vi "Config Type Def to Generic Type Defs.vi"(11 "measurement configuration":T15={"digital serial cfg file"="", "digital channel list"="7821\\PCMo 8", "master clock channel list"="7821\\PCMo 0", "output level"=-1.0, "output level units"=enum."dBFS", "output range (pk-pk)"=15.0, "load impedance"=4.0, "signal phase"=0.0, "acq sampling rate"=51200.0, "min measurement cycles"=20, "min measurement time (s)"=0.1, "min settling cycles"=0, "min settling time (s)"=0.0, "acq channel"="", "band start"=20.0, "band stop"=20000.0, "weighting filter"=enum."A-weighting", "highpass filter"=enum."DC", "lowpass filter"=enum."No filter", "sweep start frequency (Hz)"=20.0, "sweep stop frequency (Hz)"=20000.0, "number of steps"=10, "sweep profile"=enum."Logarithmic", "SNR units"=enum."dB", "THD+N units"=enum."dB", "THD units"=enum."dB", "gain units"=enum."dB", "enable regulation"=FALSE, "regulation target"=enum."THD+N Ratio", "regulation target value"=0.05, "regulation target value units"=enum."%", "regulation start level"=10.0, "regulation stop level"=70.0, "regulation number of steps"=2} {"min settling cycles" format="%#_6pHz"; "sweep start frequency (Hz)" format="%0.2f"; "acq sampling rate" format="%0.2f"}) -> (2 "regulation settings":T12={"enable regulation"=FALSE, "regulation target"=enum."THD+N Ratio", "regulation target value"=0.05, "regulation target value units"=enum."%", "regulation start level"=10.0, "regulation stop level"=70.0, "regulation number of steps"=2}, 3 "single tone settings":T1={"digital channel list"="7821\\PCMo 8", "frame clock rate"=48000.0, "number of channels"=2, "channel length"=32, "bit depth"=24, "data justification"=enum."Left Justified", "endianness"=enum."MSB First", "bit clock edge sync"=enum."Falling", "frame sync edge for channel 0"=enum."Falling", "channel 0 offset"=1, "master clock channel list"="7821\\PCMo 0", "master clock rate"=12288000.0, "enable dither"=TRUE, "logic level"=enum."3.3 V", "signal frequency"=1000.0, "output level"=-1.0, "output level units"=enum."dBFS", "output range (pk-pk)"=15.0, "load impedance"=4.0, "signal phase"=0.0, "acq sampling rate"=51200.0, "min measurement cycles"=20, "min measurement time (s)"=0.1, "min settling cycles"=0, "min settling time (s)"=0.0, "acq channel"="", "band start"=20.0, "band stop"=20000.0, "weighting filter"=enum."A-weighting", "highpass filter"=enum."DC", "lowpass filter"=enum."No filter", "SNR units"=enum."dB", "THD+N units"=enum."dB", "THD units"=enum."dB", "gain units"=enum."dB"} {"signal phase" format="%0.2f"; "master clock rate" format="%#_6pHz"; "frame clock rate" format="%#_6pHz"})   [LabVIEW 2021, in "Stepped Frequency Sweep_Class D Amplifier.lvlib"]
uses:
  Stepped Frequency Sweep_Class D Amplifier.lvlib
  Measurement Configuration.ctl
  shared/controls/digital output level units.ctl
  shared/controls/weighting filter.ctl
  shared/controls/highpass filter.ctl
  shared/controls/lowpass filter.ctl
  shared/controls/sweep profile.ctl
  shared/controls/units - snr.ctl
  shared/controls/units - ratio.ctl
  shared/controls/regulation target.ctl
  shared/controls/regulation target value units.ctl
  shared/controls/regulation settings.ctl
  shared/controls/single tone measurement settings (HW).ctl
  shared/controls/digital audio protocol/data justification.ctl
  shared/controls/digital audio protocol/endianness.ctl
  shared/controls/digital audio protocol/digital edge.ctl
  shared/controls/digital audio protocol/logic level.ctl
  shared/controls/audio controls.lvlib
  shared/digital serial gen settings/digital audio protocol controls.lvlib
panel:
  out "error out":errorcluster
  in  "error in (no error)":errorcluster
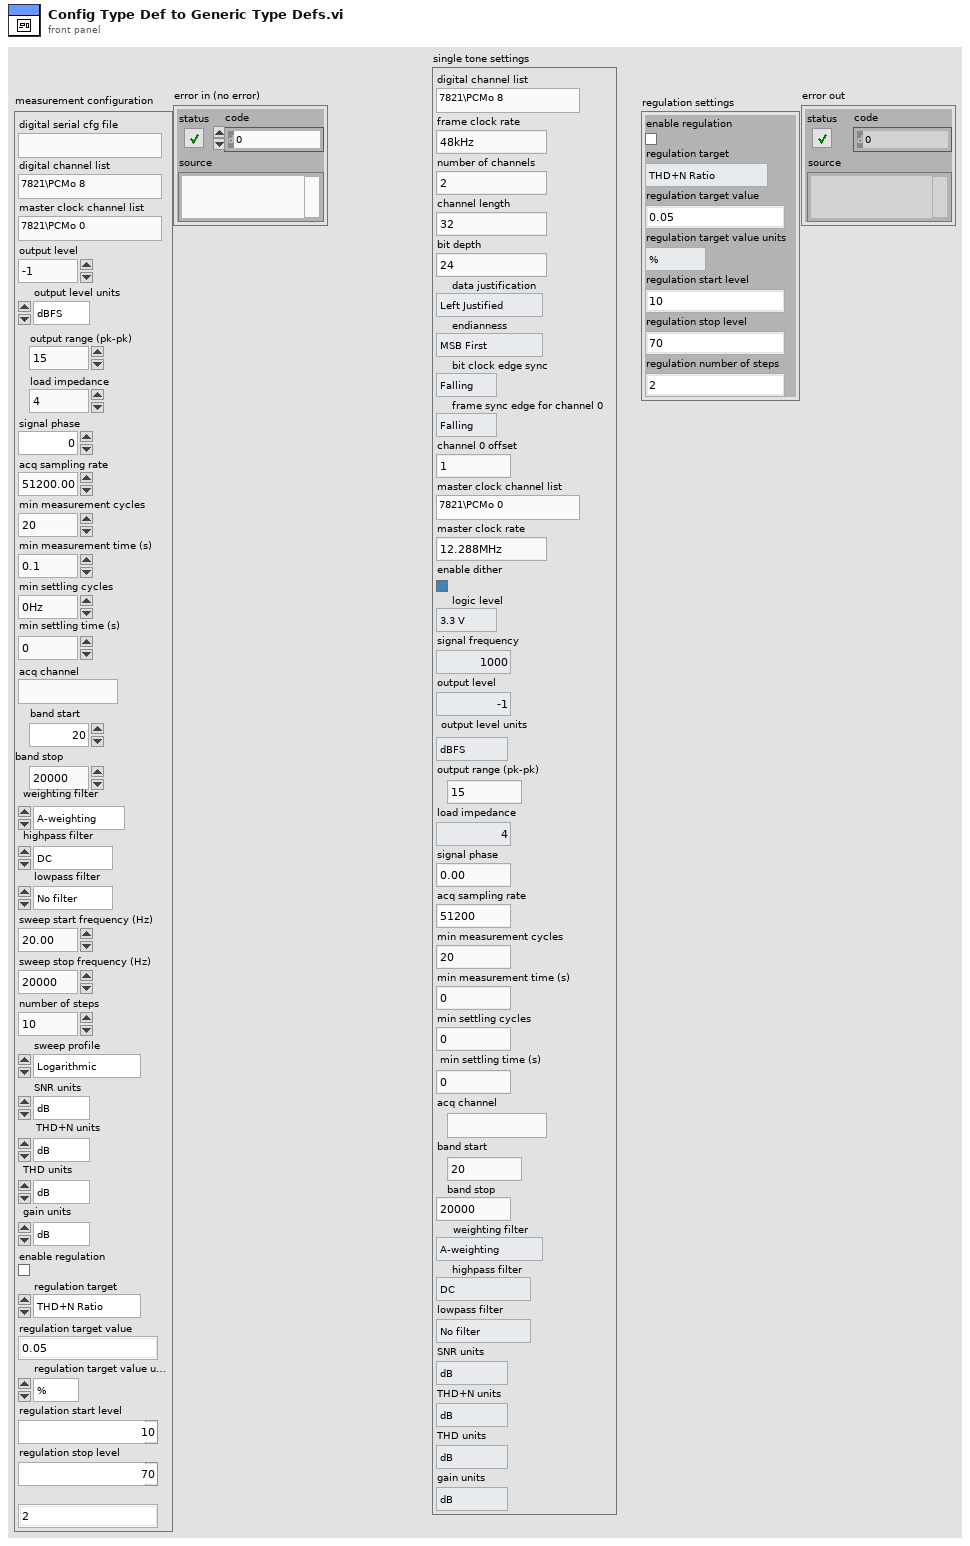
[diagram p1: front panel]
types:
  T1 = typedef "single tone measurement settings (HW).ctl" = cluster{"digital channel list":string, "frame clock rate":dbl, "number of channels":u32, "channel length":u32, "bit depth":u32, "data justification":T2, "endianness":T3, "bit clock edge sync":T4, "frame sync edge for channel 0":T4, "channel 0 offset":u32, "master clock channel list":string, "master clock rate":dbl, "enable dither":bool, "logic level":T5, "signal frequency":dbl, "output level":dbl, "output level units":T6, "output range (pk-pk)":dbl, "load impedance":dbl, "signal phase":dbl, "acq sampling rate":dbl, "min measurement cycles":u32, "min measurement time (s)":dbl, "min settling cycles":u32, "min settling time (s)":dbl, "acq channel":string, "band start":dbl, "band stop":dbl, "weighting filter":T7, "highpass filter":T8, "lowpass filter":T9, "SNR units":T10, "THD+N units":T11, "THD units":T11, "gain units":T11}
  T2 = typedef "data justification.ctl" = enum32{"Left Justified", "Right Justified"}
  T3 = typedef "endianness.ctl" = enum32{"MSB First", "LSB First"}
  T4 = typedef "digital edge.ctl" = enum32{"Rising", "Falling"}
  T5 = typedef "logic level.ctl" = enum32{"3.3 V", "1.8 V", "1.2 V"}
  T6 = typedef "audio controls.lvlib/digital output level units.ctl" = enum32{"% FS", "dBFS", "V"}
  T7 = typedef "weighting filter.ctl" = enum32{"Linear", "A-weighting", "B-weighting", "C-weighting"}
  T8 = typedef "highpass filter.ctl" = enum32{"DC", "AC"}
  T9 = typedef "lowpass filter.ctl" = enum32{"No filter", "AES17 20kHz", "AES17 40kHz"}
  T10 = typedef "audio controls.lvlib/units - snr.ctl" = enum32{"dB", "x/y"}
  T11 = typedef "audio controls.lvlib/units - ratio.ctl" = enum32{"dB", "%", "x/y"}
  T12 = typedef "regulation settings.ctl" = cluster{"enable regulation":bool, "regulation target":T13, "regulation target value":dbl, "regulation target value units":T14, "regulation start level":dbl, "regulation stop level":dbl, "regulation number of steps":u32}
  T13 = typedef "regulation target.ctl" = enum32{"THD+N Ratio", "Output Power"}
  T14 = typedef "regulation target value units.ctl" = enum32{"%", "W"}
  T15 = typedef "Stepped Frequency Sweep_Class D Amplifier.lvlib/Measurement Configuration.ctl" = cluster{"digital serial cfg file":string, "digital channel list":string, "master clock channel list":string, "output level":dbl, "output level units":T6, "output range (pk-pk)":dbl, "load impedance":dbl, "signal phase":dbl, "acq sampling rate":dbl, "min measurement cycles":u32, "min measurement time (s)":dbl, "min settling cycles":u32, "min settling time (s)":dbl, "acq channel":string, "band start":dbl, "band stop":dbl, "weighting filter":T7, "highpass filter":T8, "lowpass filter":T9, "sweep start frequency (Hz)":dbl, "sweep stop frequency (Hz)":dbl, "number of steps":u32, "sweep profile":T16, "SNR units":T10, "THD+N units":T11, "THD units":T11, "gain units":T11, "enable regulation":bool, "regulation target":T13, "regulation target value":dbl, "regulation target value units":T14, "regulation start level":dbl, "regulation stop level":dbl, "regulation number of steps":u32}
  T16 = typedef "audio controls.lvlib/sweep profile.ctl" = enum32{"Linear", "Logarithmic"}
  T17 = typedef "digital serial gen settings.ctl" = cluster{"number of channels":u32, "data justification":T18, "endianness":T19, "channel length":u32, "bit depth":u32, "frame clock rate":dbl, "bit clock edge sync":T20, "master clock rate":dbl, "Logic Level":T21, "frame sync edge for channel 0":T20, "Channel 0 Offset":u32}
  T18 = typedef "PDM Shared.lvlib/PCM Data Justification.ctl" = enum16{"Left Justified", "Right Justified"}
  T19 = typedef "PDM Shared.lvlib/PCM Bit Endianness.ctl" = enum16{"MSB First", "LSB First"}
  T20 = typedef "PDM Shared.lvlib/Digital Edge.ctl" = enum8{"Rising", "Falling"}
  T21 = typedef "PDM Acquisition Class Library.lvlib/DecoderSession.lvclass/Logic Levels.ctl" = enum16{"3.3 V", "1.8 V", "1.2 V"}
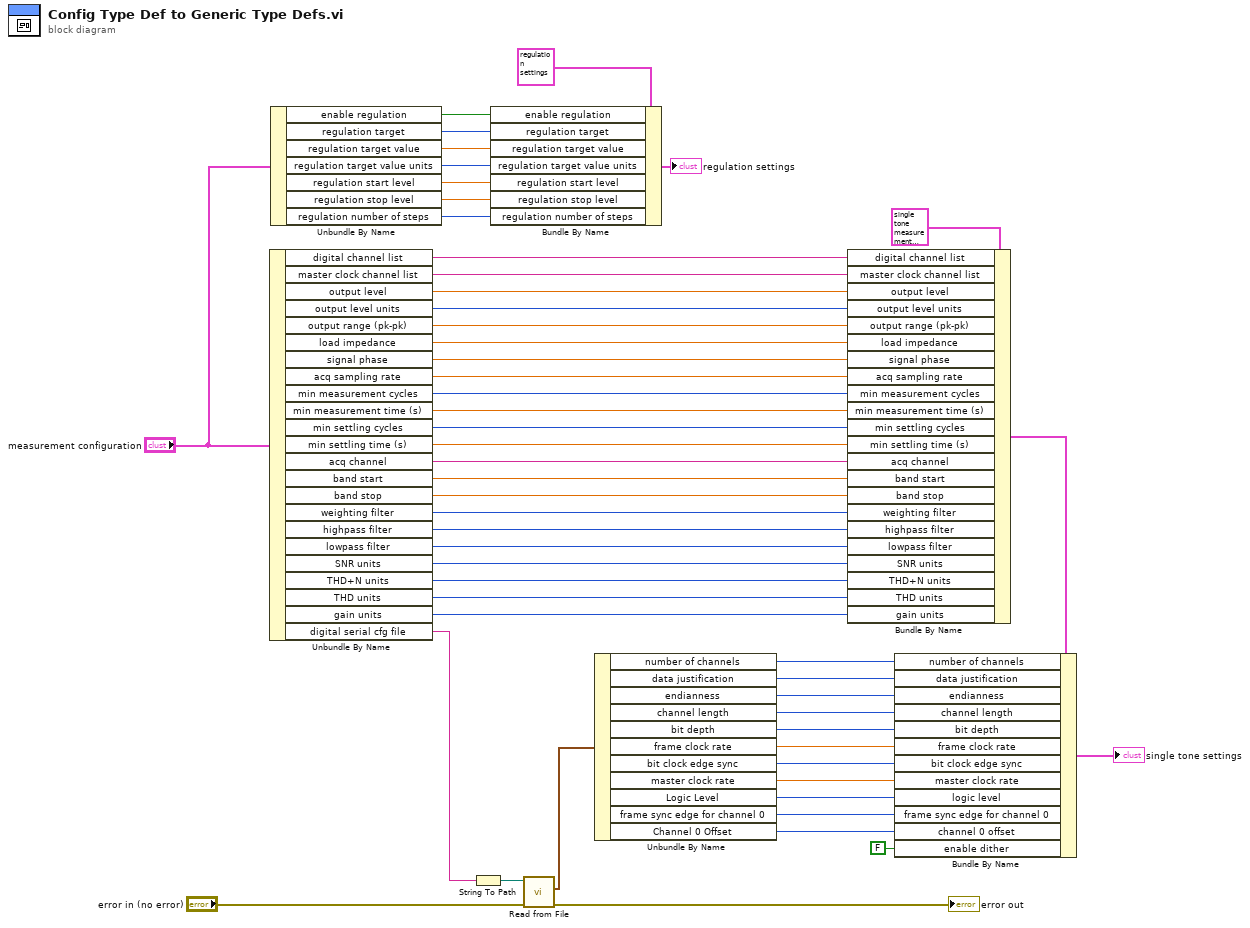
[diagram p0: block diagram]
diagram:
  n1 = Unbundle By Name("measurement configuration") -> ("digital channel list"=w42:string, "master clock channel list"=w41:string, "output level"=w21:dbl, "output level units"=w40:T6, "output range (pk-pk)"=w39:dbl, "load impedance"=w38:dbl, "signal phase"=w37:dbl, "acq sampling rate"=w36:dbl, "min measurement cycles"=w35:u32, "min measurement time (s)"=w34:dbl, "min settling cycles"=w33:u32, "min settling time (s)"=w32:dbl, "acq channel"=w31:string, "band start"=w30:dbl, "band stop"=w29:dbl, "weighting filter"=w28:T7, "highpass filter"=w27:T8, "lowpass filter"=w26:T9, "SNR units"=w25:T10, "THD+N units"=w24:T11, "THD units"=w23:T11, "gain units"=w22:T11, "digital serial cfg file"=w18:string)
  n2 = Unbundle By Name("measurement configuration") -> ("enable regulation"=w51:bool, "regulation target"=w50:T13, "regulation target value"=w49:dbl, "regulation target value units"=w48:T14, "regulation start level"=w47:dbl, "regulation stop level"=w46:dbl, "regulation number of steps"=w45:u32)
  n3 = String To Path(string=w18) -> (path=w20:path)
  n4 = Bundle By Name(cluster=T12 {"enable regulation"=FALSE, "regulation target"=enum."THD+N Ratio", "regulation target value"=0.05, "regulation target value units"=enum."%", "regulation start level"=10.0, "regulation stop level"=70.0, "regulation number of steps"=2} ("regaultion settings"), "enable regulation"=w51, "regulation target"=w50, "regulation target value"=w49, "regulation target value units"=w48, "regulation start level"=w47, "regulation stop level"=w46, "regulation number of steps"=w45) -> (→"regulation settings":T12)
  n5 = call "Read from File.vi"("error in (no error)"="error in (no error)", "file path"=w20) -> ("error out"=→"error out":errorcluster, "digital audio protocol settings"=w16:T17)  [unwired: 7 in, 1 out]
  n6 = Unbundle By Name(w16) -> ("number of channels"=w14:u32, "data justification"=w12:T18, "endianness"=w11:T19, "channel length"=w10:u32, "bit depth"=w9:u32, "frame clock rate"=w8:dbl, "bit clock edge sync"=w7:T20, "master clock rate"=w6:dbl, "Logic Level"=w5:T21, "frame sync edge for channel 0"=w4:T20, "Channel 0 Offset"=w3:u32)
  n7 = Bundle By Name(cluster=T1 {"digital channel list"="7821\\PCMo 8", "frame clock rate"=48000.0, "number of channels"=2, "channel length"=32, "bit depth"=24, "data justification"=enum."Left Justified", "endianness"=enum."MSB First", "bit clock edge sync"=enum."Falling", "frame sync edge for channel 0"=enum."Falling", "channel 0 offset"=1, "master clock channel list"="7821\\PCMo 0", "master clock rate"=12288000.0, "enable dither"=TRUE, "logic level"=enum."3.3 V", "signal frequency"=1000.0, "output level"=-1.0, "output level units"=enum."dBFS", "output range (pk-pk)"=15.0, "load impedance"=4.0, "signal phase"=0.0, "acq sampling rate"=51200.0, "min measurement cycles"=20, "min measurement time (s)"=0.1, "min settling cycles"=0, "min settling time (s)"=0.0, "acq channel"="", "band start"=20.0, "band stop"=20000.0, "weighting filter"=enum."A-weighting", "highpass filter"=enum."DC", "lowpass filter"=enum."No filter", "SNR units"=enum."dB", "THD+N units"=enum."dB", "THD units"=enum."dB", "gain units"=enum."dB"} ("measurement configuration"), "digital channel list"=w42, "master clock channel list"=w41, "output level"=w21, "output level units"=w40, "output range (pk-pk)"=w39, "load impedance"=w38, "signal phase"=w37, "acq sampling rate"=w36, "min measurement cycles"=w35, "min measurement time (s)"=w34, "min settling cycles"=w33, "min settling time (s)"=w32, "acq channel"=w31, "band start"=w30, "band stop"=w29, "weighting filter"=w28, "highpass filter"=w27, "lowpass filter"=w26, "SNR units"=w25, "THD+N units"=w24, "THD units"=w23, "gain units"=w22) -> (w15:T1)
  n8 = Bundle By Name(cluster=w15, "number of channels"=w14, "data justification"=w12, "endianness"=w11, "channel length"=w10, "bit depth"=w9, "frame clock rate"=w8, "bit clock edge sync"=w7, "master clock rate"=w6, "logic level"=w5, "frame sync edge for channel 0"=w4, "channel 0 offset"=w3, "enable dither"=FALSE) -> (→"single tone settings":T1)
